vi "Scale to Picture Rectangle.vi"(8 "Draw Area Size":T1, 9 "Length (in)":dbl, 10 "width (in)":dbl, 11 "Translation XYZ":dbl[](array[numeric])) -> (3 "offset":cluster{dbl, dbl})   [LabVIEW 2023]
uses:
  <vilib>/Utility/miscctls.llb/LVBoundsTypeDef.ctl
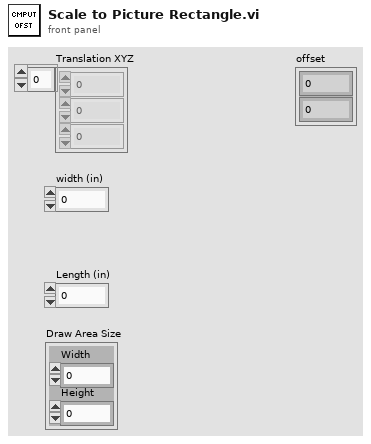
[diagram p1: front panel]
types:
  T1 = typedef "LVBoundsTypeDef.ctl" = cluster{"Width":u32, "Height":u32}
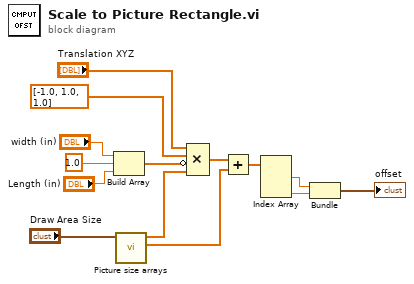
[diagram p0: block diagram]
diagram:
  n1 = Build Array("width (in)", 1.0, "Length (in)") -> (w7:dbl[])
  n2 = call "Picture size arrays.vi"("Draw Area Size"="Draw Area Size") -> ("Center"=w9:dbl[], "Size"=w14:dbl[])  [unwired: 9 in]
  n3 = Compound Arithmetic op=MULTIPLY("Translation XYZ", dbl[] [-1.0, 1.0, 1.0] ("x"), invert w7, w14) -> (w11:dbl[])
  n4 = Add(x=w11, y=w9) -> (x+y=w1:dbl[])
  n5 = Index Array(array=w1) -> (element #1=w3:dbl, element #3=w2:dbl)  [unwired: 3 in, 1 out]
  n6 = Bundle(w3, w2) -> (→"offset":cluster{dbl, dbl})  [unwired: 1 in]
